vi "PH_Beckhoff.ProcCases.vi"(0 "i ref in":refnum<vi>, 1 "selector":string, 2 "Data":T1, 3 "call cluster":T2={"Object"="", "Selector"="", "CallType"=enum."synchronous", "Async Object"="", "Async Selector"="", "Data Descriptor"="", "Data"=[], "Error #"=0, "Expire"=0}, 5 "error in (no error)":errorcluster) -> (14 "i ref out":refnum<vi>, 17 "answer cluster":T2={"Object"="", "Selector"="", "CallType"=enum."synchronous", "Async Object"="", "Async Selector"="", "Data Descriptor"="", "Data"=[], "Error #"=0, "Expire"=0}, 19 "error out":errorcluster)   [LabVIEW 2014, in "PH_Beckhoff.lvlib"]
doc: "This method is called by a process from within the default case in the event loop. The methods of a class that are linked to events will be called from THIS method. Add your code here."
uses:
  PH_Beckhoff.lvlib
  CS_Core/CSSystem/CoreDefs/CoreDefs.call_type.ctl
  CS_Core/BaseProcess/BaseProcess.descriptor string definition.ctl
  CS_Core/CSSystem/CoreDefs/CoreDefs.rawDataType.ctl
  CS_Core/CSSystem/CoreLib/CoreLib.string 2 byte array.vi
  CS_Core/BaseProcess/BaseProcess.lvlib
  CS_Core/CSSystem/CoreLib/CoreLib.lvlib
  PH_Basics/PH_Class/PH_Class.lvlib
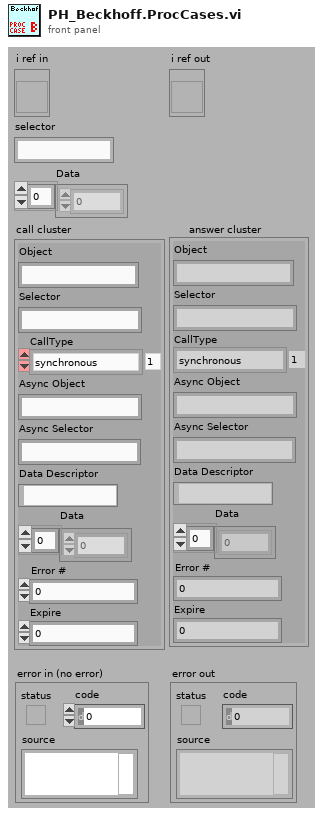
[diagram p1: front panel]
types:
  T1 = typedef "CoreDefs.rawDataType.ctl" = i8[]
  T2 = typedef "CoreDefs.call_type.ctl" = cluster{"Object":string, "Selector":string, "CallType":enum16{"simple", "synchronous", "asynchronous"}, "Async Object":string, "Async Selector":string, "Data Descriptor":T3, "Data":T1, "Error #":i32, "Expire":u32}
  T3 = typedef "BaseProcess.lvlib/BaseProcess.descriptor string definition.ctl" = string
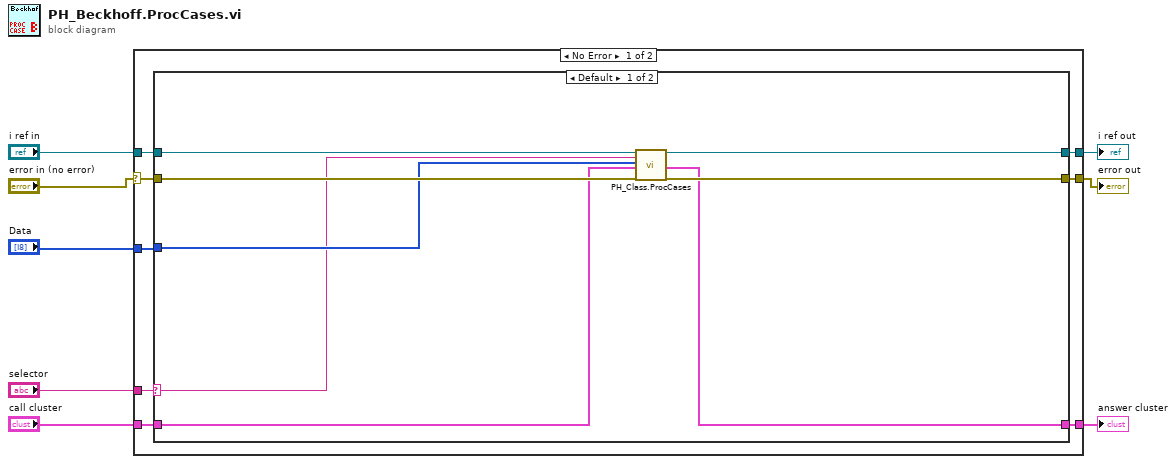
[diagram p0: block diagram]
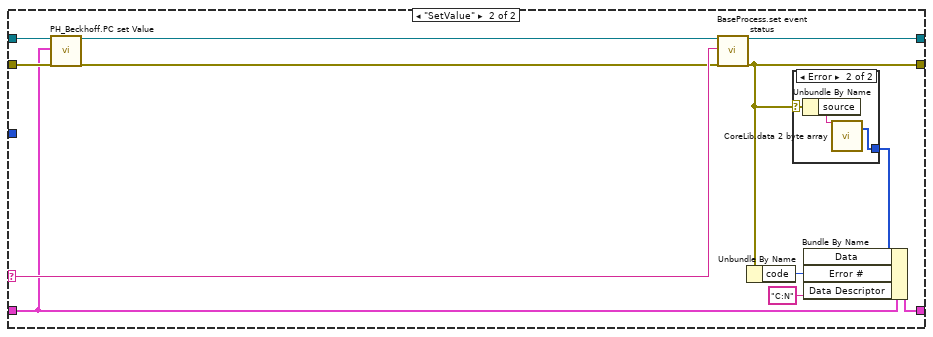
[diagram p2: hidden frame]
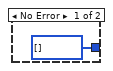
[diagram p3: hidden frame]
diagram:
  n1 = case shown="No Error" "error in (no error)" {
    selector: "error in (no error)" -> [w9 w41]
    tunnel: "selector" -> [w16 _]
    tunnel: [w15 w42] -> w7
    tunnel: "Data" -> [w14 _]
    tunnel: "call cluster" -> [w13 w42]
    tunnel: "i ref in" -> [w12 w43]
    tunnel: [w11 w43] -> w3
    tunnel: [w10 w41] -> w2
    frame No Error {
      n2 = case shown="Default" w16 {
        selector: w16 -> [w18 w30]
        tunnel: w14 -> [w19 _]
        tunnel: w12 -> [w17 w27]
        tunnel: [w24 w32] -> w11
        tunnel: w13 -> [w20 w25]
        tunnel: [w21 w35] -> w15
        tunnel: w9 -> [w23 w26]
        tunnel: [w22 w33] -> w10
        frame Default {
          n3 = call "PH_Class.ProcCases.vi"("i ref in"=w17, "selector"=w18, "Data"=w19, "call cluster"=w20, "error in (no error)"=w23) -> ("i ref out"=w24:refnum<vi>, "answer cluster"=w21:T2, "error out"=w22:errorcluster)  [unwired: 12 in]
        }
        frame "SetValue" {
          n4 = call "PH_Beckhoff.PC set Value.vi"("i ref in"=w27, "call cluster"=w25, "error in"=w26) -> ("i ref out"=w28:refnum<vi>, "error out"=w29:errorcluster)  [unwired: 15 in]
          n5 = call "BaseProcess.set event status.vi"("i ref in"=w28, "EventStatus"=w30, "error in (no error)"=w29) -> ("i ref out"=w32:refnum<vi>, "error out"=w33:errorcluster)  [unwired: 14 in, 1 out]
          n6 = Unbundle By Name(w33) -> ("code"=w36:i32)
          n7 = case shown="Error" w33 {
            selector: w33 -> [_ w40]
            tunnel: [T1 [] ("byteArray out") w39] -> w34
            frame No Error {
            }
            frame Error {
              n8 = Unbundle By Name(w40) -> ("source"=w38:string)
              n9 = call-poly "CoreLib.data 2 byte array.vi"("string"=w38) -> ("byteArray out"=w39:T1)  [unwired: 18 in]
            }
          }
          n10 = Bundle By Name(cluster=w25, "Data"=w34, "Error #"=w36, "Data Descriptor"="C:N") -> (w35:T2)
        }
      }
    }
    frame Error {
    }
  }
  "answer cluster" <- w7
  "i ref out" <- w3
  "error out" <- w2
